vi "FTP自动升级更新main.vi"() -> ()   [LabVIEW 2016, in "数据传输系统-02.lvlib" / "自动更新.lvlib"]
uses:
  <vilib>/FTP/NI_FTP.lvlib
panel:
  out "有新版本":bool
  out "最新版本获取进度":u8(slide) scale=0.0..100.0
  # "版本获取中，请稍后！"
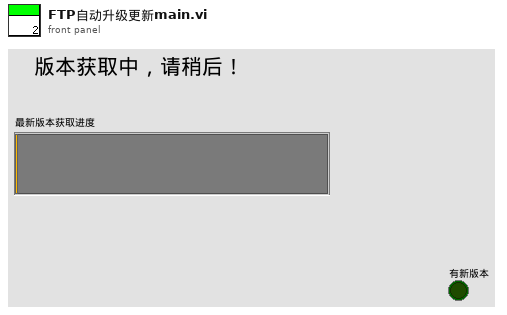
[diagram p1: front panel]
types:
  T1 = enum16{"get version information", "get success", "contact", "over"}
  T2 = cluster{"网络灯":bool, "接收中":bool, "已接收百分比":u8, "接收成功次数":dbl, "当前步骤":enum16{"init", "receivehead", "receivecontent", "receivesuccess", "over"}, "文件名":string, "error out":errorcluster}
  T3 = enum16{"open", "replace", "create", "open or create", "replace or create", "replace or create with confirmation"}
  T4 = cluster{"主机":string, "用户":string, "密码":string, "远程路径":string, "下载文件名":string, "软件版本":string}
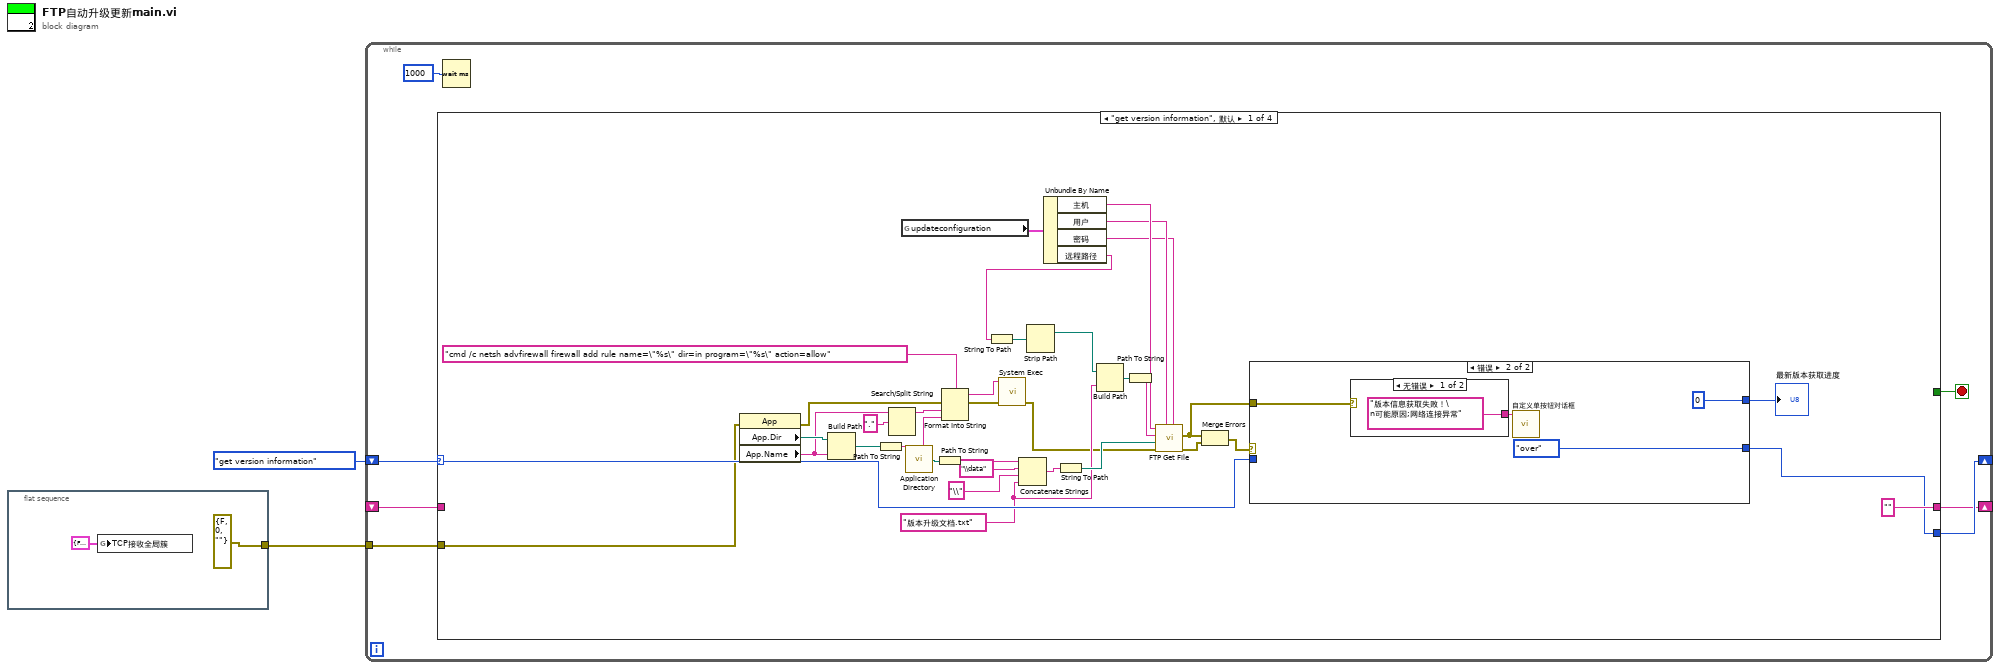
[diagram p0: block diagram]
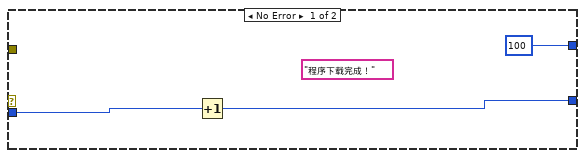
[diagram p2: hidden frame]
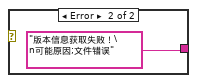
[diagram p3: hidden frame]
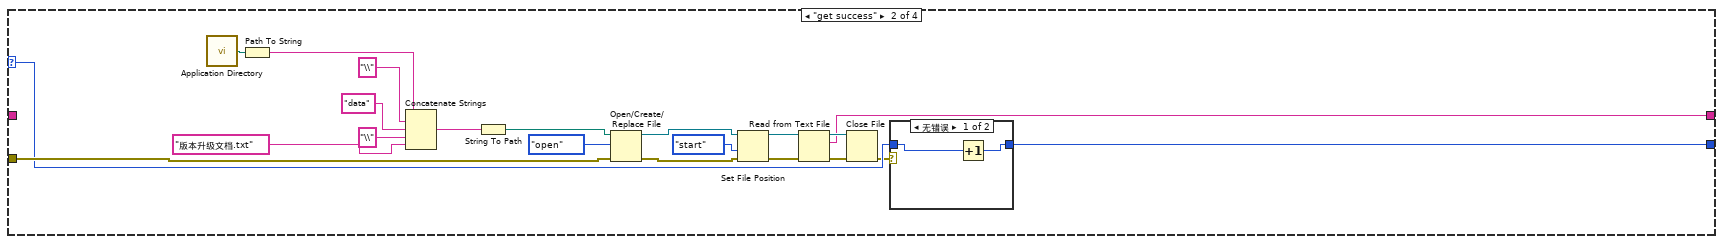
[diagram p4: hidden frame]
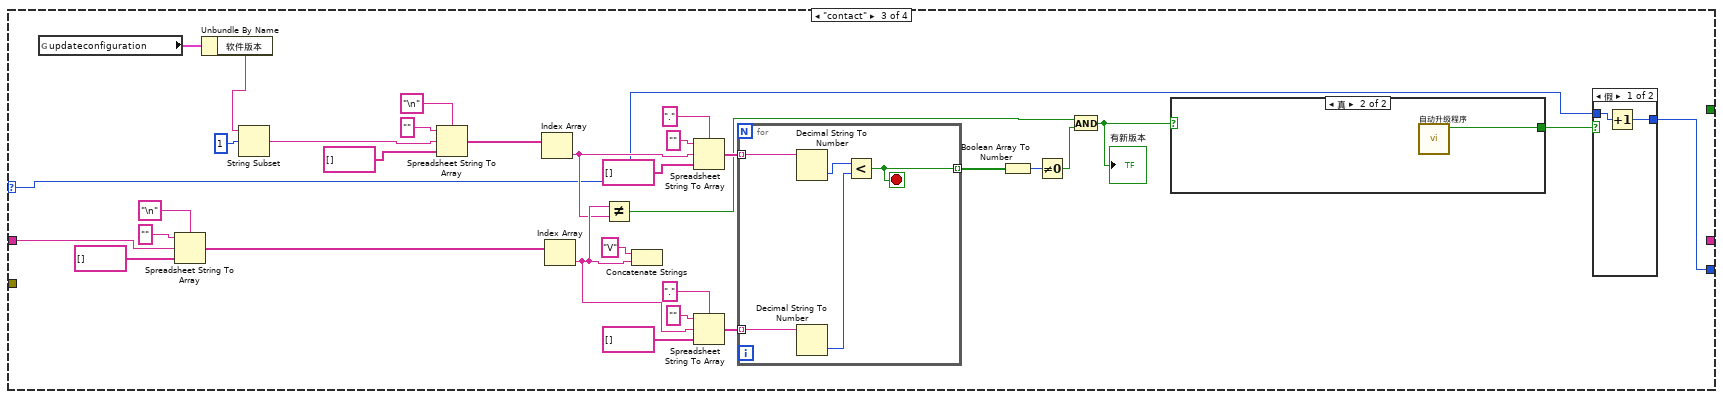
[diagram p6: hidden frame]
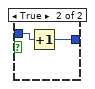
[diagram p7: hidden frame]
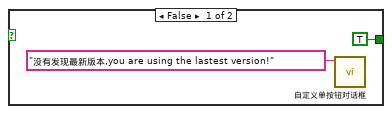
[diagram p8: hidden frame]
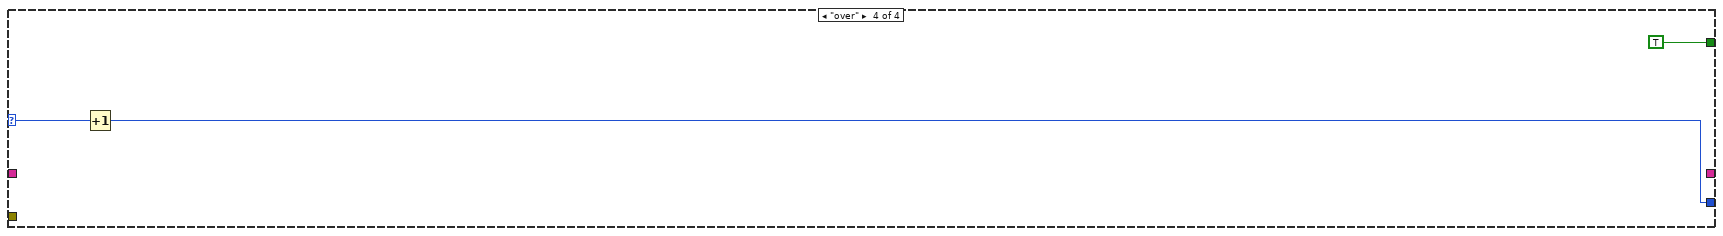
[diagram p9: hidden frame]
diagram:
  n1 = flat-sequence {
    tunnel: [errorcluster {"status"=FALSE, "code"=0, "source"=""} ("错误常量")] -> w1
    frame #0 {
      n2 = global write "全局变量1.vi" "TCP接收全局簇"(T2 {"网络灯"=FALSE, "接收中"=FALSE, "已接收百分比"=0, "接收成功次数"=0.0, "当前步骤"=enum."init", "文件名"="", "error out"={"status"=FALSE, "code"=0, "source"=""}} ("TCP接收全局簇")) -> ()
    }
  }
  n3 = while {
    shift-right: [w9] -> _
    shift-left: T1."get version information" -> [w10]
    tunnel: w1 -> [w8]
    shift-right: [w7] -> _
    shift-left: _ -> [w6]
    stop <- w5 stop-if-true
    n4 = case shown="\"get version information\", 默认" w10 {
      selector: w10 -> [w36 w63 w83 w125]
      tunnel: [w35 w62 w82 w124] -> w9
      tunnel: w8 -> [w12 w64 _ _]
      tunnel: ["" w56 _ _] -> w7
      tunnel: w6 -> [_ _ w86 _]
      tunnel: [_ _ _ TRUE] -> w5
      frame "get version information", Default {
        w26 = "版本升级文档.txt"
        n5 = property class="App"(error in=w12) -> (error out=w17:errorcluster, "App.Dir"=w23:path, "App.Name"=w19:string)  [unwired: 1 in, 1 out]
        n6 = Build Path(base path=w23, name or relative path=w19) -> (appended path=w22:path)
        n7 = Path To String(path=w22) -> (string=w21:string)
        n8 = Search/Split String(string=w19, search string/char (-)="." ("搜索字符串/字符(-)")) -> (substring before match=w18:string)  [unwired: 1 in, 2 out]
        n9 = global read "update全局.vi" "updateconfiguration"() -> (w34:T4)
        n10 = call <vilib>:"Application Directory.vi"() -> ("Application Directory"=w43:path)
        n11 = Path To String(path=w43) -> (string=w45:string)
        n12 = Format Into String(format string="cmd /c netsh advfirewall firewall add rule name=\"%s\" dir=in program=\"%s\" action=allow" ("command line"), error in=w17, w18, w21) -> (resulting string=w14:string, error out=w16:errorcluster)  [unwired: 1 in]
        n13 = call <vilib>:"System Exec.vi"("error in (no error)"=w16, "command line"=w14) -> ("error out"=w13:errorcluster)  [unwired: 6 in, 3 out]
        n14 = Concatenate Strings(w45, "\\data" ("字符串"), "\\" ("字符串"), w26) -> (w42:string)
        n15 = Unbundle By Name(w34) -> ("主机"=w33:string, "用户"=w32:string, "密码"=w31:string, "远程路径"=w27:string)
        n16 = String To Path(string=w27) -> (path=w29:path)
        n17 = Strip Path(path=w29) -> (stripped path=w28:path)  [unwired: 1 out]
        n18 = String To Path(string=w42) -> (path=w41:path)
        n19 = Build Path(base path=w28, name or relative path=w26) -> (appended path=w25:path)
        n20 = Path To String(path=w25) -> (string=w24:string)
        n21 = call <vilib>:"FTP Get File.vi"("password"=w31, "user"=w32, "error in (no error)"=w13, "local path"=w41, "remote path"=w24, "host"=w33) -> ("error out"=w40:errorcluster, "file error"=w38:errorcluster)  [unwired: 4 in]
        n22 = Merge Errors(w38, w40) -> (w39:errorcluster)
        n23 = case shown="错误" w39 {
          tunnel: w38 -> [_ w52]
          tunnel: [u8 100 ("y") u8 0 ("y")] -> w37
          tunnel: [w48 T1."over"] -> w35
          tunnel: w36 -> [w47 _]
          frame No Error {
            (unwired) "程序下载完成！"
            n24 = Increment(x=w47) -> (x+1=w48:T1)
          }
          frame Error {
            n25 = case shown="无错误" w52 {
              tunnel: ["版本信息获取失败！\n可能原因;网络连接异常" "版本信息获取失败！\n可能原因;文件错误"] -> w53
              frame No Error {
              }
              frame Error {
              }
            }
            n26 = call "自定义单按钮对话框.vi"("消息"=w53) -> ()  [unwired: 11 in]
          }
        }
        "最新版本获取进度" <- w37
      }
      frame "get success" {
        n27 = call <vilib>:"Application Directory.vi"() -> ("Application Directory"=w69:path)
        n28 = Path To String(path=w69) -> (string=w72:string)
        n29 = Concatenate Strings(w72, "\\" ("字符串"), "data" ("字符串"), "\\" ("字符串"), "版本升级文档.txt" ("字符串")) -> (w66:string)
        n30 = String To Path(string=w66) -> (path=w65:path)
        n31 = Open/Create/Replace File(file path (use dialog)=w65, error in=w64, operation (0:open)=T3."open" ("操作(0:open)")) -> (refnum out=w75:refnum<file>, error out=w74:errorcluster)  [unwired: 3 in, 1 out]
        n32 = Set File Position(refnum=w75, from (0:start)=enum16{"start", "end", "current"}."start" ("自（0:起始）"), error in=w74) -> (refnum out=w60:refnum<file>, error out=w59:errorcluster)  [unwired: 1 in]
        n33 = Read from Text File(file (use dialog)=w60, error in=w59) -> (refnum out=w61:refnum<file>, text=w56:string, error out=w58:errorcluster)  [unwired: 2 in, 1 out]
        n34 = Close File(refnum=w61, error in=w58) -> (error out=w57:errorcluster)  [unwired: 1 out]
        n35 = case shown="无错误" w57 {
          tunnel: w63 -> [w78 w79]
          tunnel: [w77 w79] -> w62
          frame No Error {
            n36 = Increment(x=w78) -> (x+1=w77:T1)
          }
          frame Error {
          }
        }
      }
      frame "contact" {
        n37 = global read "update全局.vi" "updateconfiguration"() -> (w81:T4)
        n38 = Spreadsheet String To Array(delimiter (Tab)="\n" ("分隔符(Tab)"), format string="" ("格式字符串"), spreadsheet string=w86, array type (2D Dbl)=string[] []) -> (array=w107:string[])
        n39 = Unbundle By Name(w81) -> ("软件版本"=w80:string)
        n40 = String Subset(string=w80, offset (0)=1 ("偏移量(0)")) -> (substring=w99:string)  [unwired: 1 in]
        n41 = Spreadsheet String To Array(delimiter (Tab)="\n" ("分隔符(Tab)"), format string="" ("格式字符串"), spreadsheet string=w99, array type (2D Dbl)=string[] []) -> (array=w98:string[])
        n42 = Index Array(array=w98) -> (element=w89:string)  [unwired: 1 in]
        n43 = Index Array(array=w107) -> (element=w90:string)  [unwired: 1 in]
        n44 = Not Equal?(x=w90, y=w89) -> (x != y?=w87:bool)
        n45 = Concatenate Strings("V" ("字符串"), w90) -> ()  [unwired: 1 out]
        n46 = Spreadsheet String To Array(delimiter (Tab)="." ("分隔符(Tab)"), format string="" ("格式字符串"), spreadsheet string=w89, array type (2D Dbl)=string[] []) -> (array=w93:string[])
        n47 = Spreadsheet String To Array(delimiter (Tab)="." ("分隔符(Tab)"), format string="" ("格式字符串"), spreadsheet string=w90, array type (2D Dbl)=string[] []) -> (array=w94:string[])
        n48 = for {
          tunnel: w94 -> [w121] mode=indexing
          tunnel: w93 -> [w123] mode=indexing
          tunnel: [w122] -> w92 mode=indexing
          stop <- w122 stop-if-true
          n49 = Decimal String To Number(string=w123) -> (number=w120:i32)  [unwired: 2 in, 1 out]
          n50 = Decimal String To Number(string=w121) -> (number=w119:i32)  [unwired: 2 in, 1 out]
          n51 = Less?(x=w120, y=w119) -> (x < y?=w122:bool)
        }
        n52 = Boolean Array To Number(Boolean array=w92) -> (number=w91:u32)
        n53 = Not Equal To 0?(x=w91) -> (x != 0?=w88:bool)
        n54 = And(x=w87, y=w88) -> (x .and. y?=w85:bool)
        "有新版本" <- w85
        n55 = case shown="真" w85 {
          tunnel: [TRUE ("确定") w118] -> w84
          frame False {
            n56 = call "自定义单按钮对话框.vi"("消息"="没有发现最新版本,you are using the lastest version!") -> ()  [unwired: 11 in]
          }
          frame True {
            n57 = call "自动升级程序.vi"() -> ("确定"=w118:bool)  [unwired: 10 in, 1 out]
          }
        }
        n58 = case shown="假" w84 {
          tunnel: w83 -> [w113 w115]
          tunnel: [w112 w114] -> w82
          frame False {
            n59 = Increment(x=w113) -> (x+1=w112:T1)
          }
          frame True {
            n60 = Increment(x=w115) -> (x+1=w114:T1)
          }
        }
      }
      frame "over" {
        n61 = Increment(x=w125) -> (x+1=w124:T1)
      }
    }
    n62 = Wait (ms)(milliseconds to wait=u32 1000 ("等待时间（毫秒）")) -> ()  [unwired: 1 out]
  }
